vi "approach.vi"(8 "error in (no error)":errorcluster, 11 "Input":string="f") -> (0 "error out":errorcluster, 3 "Output":string="approached")   [LabVIEW 2014]
uses:
  <userlib>/Nanonis Prog Interface V5/Nanonis Prog Interface.lvlib
panel:
  out "testing?":bool
  out "size(s)":i32=1
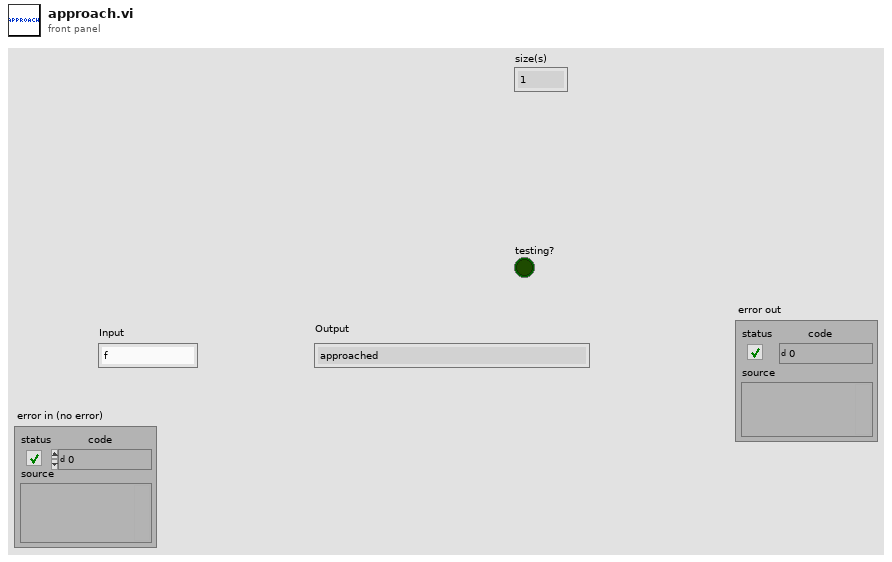
[diagram p1: front panel]
types:
  T1 = enum8{"Group 1", "Group 2", "Group 3", "Group 4", "Group 5", "Group 6"}
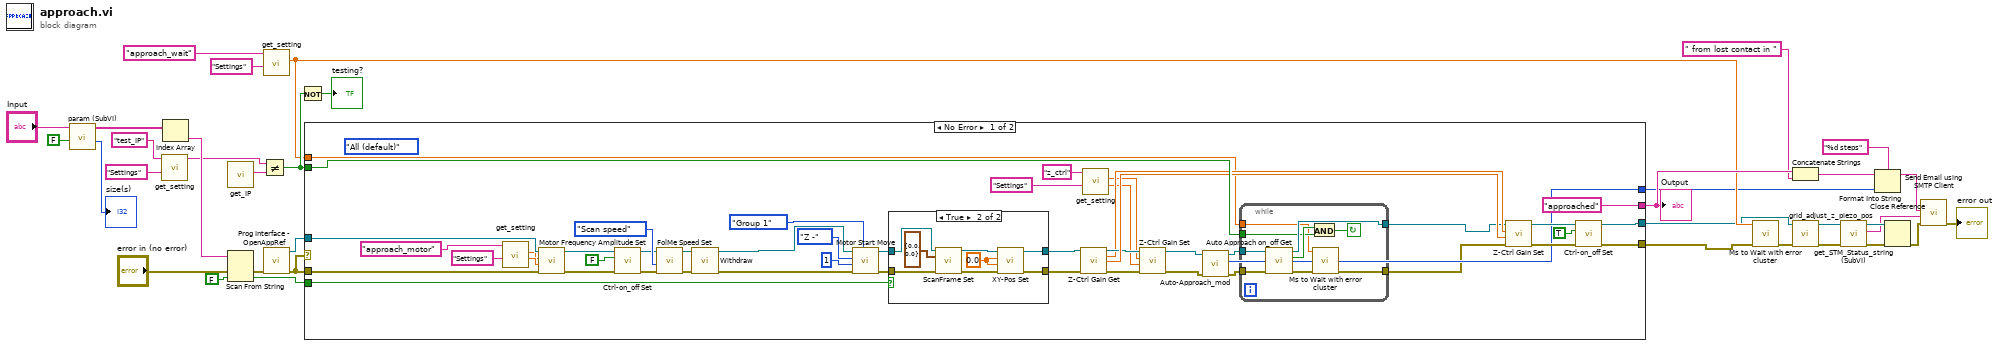
[diagram p0: block diagram]
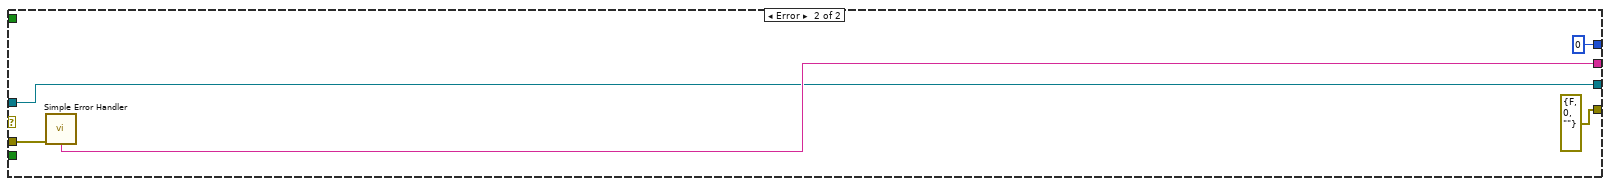
[diagram p3: hidden frame]
diagram:
  n1 = call <userlib>:"param (SubVI).vi"("Numeric"=FALSE, "Input"="Input") -> ("num"=→"size(s)":i32, "Array"=w26:string[])  [unwired: 7 in, 1 out]
  n2 = call "get_setting.vi"("section"="Settings", "key"="test_IP") -> ("value"=w10:string)  [unwired: 5 in, 4 out]
  n3 = Index Array(array=w26) -> (element=w25:string)  [unwired: 1 in]
  n4 = call "get_IP.vi"() -> ("IP address"=w30:string)  [unwired: 11 in]
  n5 = Scan From String(input string=w25, error in="error in (no error)", default 1=FALSE) -> (error out=w23:errorcluster, output 1=w21:bool)  [unwired: 2 in, 2 out]
  n6 = Not Equal?(x=w10, y=w30) -> (x != y?=w28:bool)
  n7 = call "get_setting.vi"("section"="Settings", "key"="approach_wait") -> ("output 1"=w7:dbl)  [unwired: 5 in, 4 out]
  n8 = call <userlib>:"Prog Interface - OpenAppRef.vi"("Error in (no error)"=w23) -> ("Error out"=w27:errorcluster, "Application reference"=w34:refnum<vi>)  [unwired: 5 in]
  n9 = Not(x=w28) -> (.not. x?=→"testing?":bool)
  n10 = case shown="No Error" w27 {
    tunnel: w34 -> [w59 w104]
    tunnel: w27 -> [w56 w107]
    tunnel: [w78 errorcluster {"status"=FALSE, "code"=0, "source"=""} ("error out")] -> w5
    tunnel: ["approached" ("initial string") w106] -> w19
    tunnel: [w77 w104] -> w6
    tunnel: w28 -> [w76 _]
    tunnel: w21 -> [w68 _]
    tunnel: w7 -> [w50 _]
    tunnel: [w39 0 ("steps taken")] -> w1
    frame No Error {
      (unwired) enum16{"All (default)", "X", "Y", "Z"}."All (default)" ("Axis (All)")
      n11 = call "get_setting.vi"("section"="Settings", "key"="approach_motor") -> ("output 2"=w47:dbl, "output 1"=w46:dbl)  [unwired: 5 in, 3 out]
      n12 = call <userlib>:"Motor Frequency Amplitude Set.vi"("Error in (no error)"=w56, "Amplitude (V) (NaN=no change)"=w47, "Frequency (Hz) (NaN=no change)"=w46, "Application ref in"=w59) -> ("Error out"=w57:errorcluster, "Application ref out"=w58:refnum<vi>)  [unwired: 6 in]
      n13 = call <userlib>:"Ctrl-on_off Set.vi"("error in (no error)"=w57, "Z Controller ON/OFF"=FALSE, "Application ref in"=w58) -> ("error out"=w60:errorcluster, "Application ref out"=w55:refnum<vi>)  [unwired: 7 in]
      n14 = call <userlib>:"FolMe Speed Set.vi"("error in (no error)"=w60, "Speed Setting (Custom)"=enum32{"Scan speed", "Custom speed"}."Scan speed", "Application ref in"=w55) -> ("error out"=w81:errorcluster, "Application ref out"=w82:refnum<vi>)  [unwired: 5 in]
      n15 = call <userlib>:"Withdraw.vi"("Error in (no error)"=w81, "Application ref in"=w82) -> ("Error out"=w44:errorcluster, "Application ref out"=w45:refnum<vi>)  [unwired: 8 in]
      n16 = call <userlib>:"Motor Start Move.vi"("Group"=T1."Group 1", "Error in (no error)"=w44, "Number of steps"=u16 1, "Direction"=enum16{"X +", "X -", "Y +", "Y -", "Z +", "Z -"}."Z -", "Application ref in"=w45) -> ("Error out"=w66:errorcluster, "Application ref out"=w67:refnum<vi>)  [unwired: 4 in]
      n17 = case shown="True" w68 {
        tunnel: w67 -> [w84 w93]
        tunnel: w66 -> [w85 w92]
        tunnel: [w84 w87] -> w62
        tunnel: [w85 w86] -> w61
        frame False {
        }
        frame True {
          w88 = sgl 0.0 ("X (m)")
          n18 = call <userlib>:"ScanFrame Set.vi"("Application ref in"=w93, "Center coordinates (m)"=cluster{"Xc":sgl, "Yc":sgl} {"Xc"=0.0, "Yc"=0.0}, "error in (no error)"=w92) -> ("Application ref out"=w89:refnum<vi>, "error out"=w90:errorcluster)  [unwired: 11 in]
          n19 = call <userlib>:"XY-Pos Set.vi"("error in (no error)"=w90, "Y (m)"=w88, "X (m)"=w88, "Application ref in"=w89) -> ("error out"=w86:errorcluster, "Application ref out"=w87:refnum<vi>)  [unwired: 4 in]
        }
      }
      n20 = call <userlib>:"Z-Ctrl Gain Get.vi"("Application ref in"=w62, "error in (no error)"=w61) -> ("Application ref out"=w74:refnum<vi>, "P-gain"=w73:sgl, "Time constant (s)"=w75:sgl, "error out"=w72:errorcluster)  [unwired: 9 in, 1 out]
      n21 = call "get_setting.vi"("section"="Settings", "key"="z_ctrl") -> ("output 2"=w51:dbl, "output 1"=w52:dbl)  [unwired: 5 in, 3 out]
      n22 = call <userlib>:"Z-Ctrl Gain Set.vi"("error in (no error)"=w72, "Time constant (s)"=w51, "P-gain"=w52, "Application ref in"=w74) -> ("error out"=w41:errorcluster, "Application ref out"=w40:refnum<vi>)  [unwired: 5 in]
      n23 = call "Auto-Approach_mod.vi"("Error in"=w41, "Application reference"=w40) -> ("error out"=w42:errorcluster, "steps taken"=w39:i32, "Application ref out"=w43:refnum<vi>)  [unwired: 4 in, 1 out]
      n24 = while {
        tunnel: w43 -> [w101]
        tunnel: [w100] -> w38
        tunnel: w42 -> [w99]
        tunnel: [w98] -> w37
        tunnel: w76 -> [w95]
        tunnel: w50 -> [w94]
        stop <- w96 continue-if-true
        n25 = call <userlib>:"Auto Approach on_off Get.vi"("Error in (no error)"=w99, "Application ref in"=w101) -> ("Error out"=w102:errorcluster, "Auto approach on/off status"=w97:bool, "Application ref out"=w100:refnum<vi>)  [unwired: 5 in]
        n26 = And(x=w97, y=w95) -> (x .and. y?=w96:bool)
        n27 = call <userlib>:"Ms to Wait with error cluster.vi"("error in (no error)"=w102, "milliseconds to wait"=w94) -> ("error out"=w98:errorcluster)  [unwired: 4 in, 1 out]
      }
      n28 = call <userlib>:"Z-Ctrl Gain Set.vi"("error in (no error)"=w37, "Time constant (s)"=w75, "P-gain"=w73, "Application ref in"=w38) -> ("error out"=w69:errorcluster, "Application ref out"=w71:refnum<vi>)  [unwired: 5 in]
      n29 = call <userlib>:"Ctrl-on_off Set.vi"("error in (no error)"=w69, "Z Controller ON/OFF"=TRUE, "Application ref in"=w71) -> ("error out"=w78:errorcluster, "Application ref out"=w77:refnum<vi>)  [unwired: 7 in]
    }
    frame Error {
      n30 = call <vilib>:"Simple Error Handler.vi"("error in (no error)"=w107) -> ("message"=w106:string)  [unwired: 4 in, 4 out]
    }
  }
  "Output" <- w19
  n31 = call <userlib>:"Ms to Wait with error cluster.vi"("error in (no error)"=w5, "milliseconds to wait"=w7) -> ("error out"=w14:errorcluster)  [unwired: 4 in, 1 out]
  n32 = Concatenate Strings(w19, " from lost contact in " ("string")) -> (w4:string)
  n33 = call "grid_adjust_z_piezo_pos.vi"("Error in (no error)"=w14, "Application ref in"=w6) -> ("Error out"=w16:errorcluster, "Application ref out"=w15:refnum<vi>)  [unwired: 8 in]
  n34 = call "get_STM_Status_string (SubVI).vi"("error in (no error)"=w16, "Application in"=w15) -> ("error out"=w31:errorcluster, "JSON string"=w20:string, "Application out"=w32:refnum<vi>)  [unwired: 7 in]
  n35 = Format Into String(format string="%d steps", initial string=w4, w1) -> (resulting string=w3:string)  [unwired: 1 in, 1 out]
  n36 = Close Reference(reference=w32, error in (no error)=w31) -> (error out=w18:errorcluster)
  n37 = call "Send Email using SMTP Client.vi"("error in (no error)"=w18, "Message"=w20, "subject"=w3) -> ("error out"=→"error out":errorcluster)  [unwired: 8 in]
